vi "Execute Network Operation.vi"(7 "Operation":T1, 8 "error in (no error)":errorcluster, 10 "Message":string, 11 "Listener In.lvclass":refnum<class "Listener.lvclass">) -> (0 "error out":errorcluster, 3 "Listener Out.lvclass":refnum<class "Listener.lvclass">)   [LabVIEW 2023, in "Listener.lvclass"]
doc: "Reads/Writes data using the specified protocol.\nInput: \nListener Object\nMessage: The \"packet\" which will be sent through the selected protocol\nOpeartion: Read/Write operation on the specified protocol"
uses:
  Listener.lvclass
  Protocols.lvlib
  Constants.vi
  ListenerClassControls/Operation.ctl
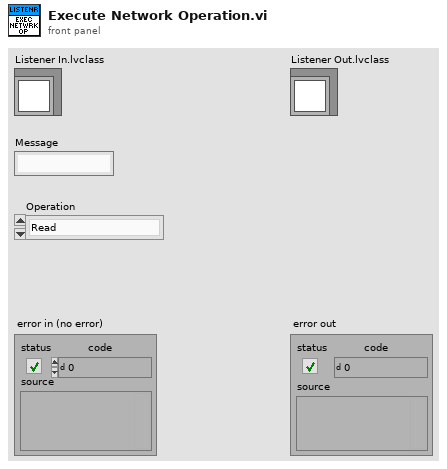
[diagram p1: front panel]
types:
  T1 = typedef "Listener.lvclass/Operation.ctl" = enum16{"Read", "Write"}
  T2 = enum16{"Standard", "Buffered", "CRLF", "Immediate"}
  T3 = typedef "Listener.lvclass/Protocol.ctl" = enum16{"RS-XXX", "AK RS-XXX", "VISA", "TCPIP", "AK TCPIP", "UDP", "GPIB ConvBox"}
  T4 = typedef "Listener.lvclass/UDP Data Structure.ctl" = cluster{"UDP connection ID":refnum<k16>, "Local Address":string, "Local Port":u16, "Target IP Address":string, "Target Port":u16, "Data":string}
  T5 = typedef "Listener.lvclass/TCP Data Structure.ctl" = cluster{"TCP|IP connection ID":refnum<k5>, "IP Address":string, "Port":u16, "Data":string}
  T6 = typedef "Listener.lvclass/AK TCP Data Structure.ctl" = cluster{"TCP|IP connection ID":refnum<k5>, "IP Address":string, "Port":u16, "Data":string, "Current Command Code":string}
  T7 = typedef "Listener.lvclass/VISA Data Structure.ctl" = cluster{"Data Length":u32, "Data":string}
  T8 = typedef "Listener.lvclass/RS-xxx Data Structure.ctl" = cluster{"Virtual COM Port Settings 1":cluster{"Port":string, "Baud Rate":u32, "Data Bits":u16, "Parity":enum16{"None", "Odd", "Even", "Mark", "Space"}, "Stop Bits":u16, "Flow Control":u16, "XON":enum16{"NUL", "SOH", "STX", "ETX", "EOT", "ENQ", "ACK", "BEL", "BS", "HT", "LF", "VT", "FF", "CR", "SO", "SI", "DLE", "DC1", "DC2", "DC3", "DC4", "NAK", "SYN", "ETB", "CAN", "EM", "SUB", "ESC", "FS", "GS", "RS", "US", "SP", "!", "\"", "#", "$", "%", "&", "'", "(", ")", "*", "+", ",", "- (-)", ".", "/", "0", "1", "2", "3", "4", "5", "6", "7", "8", "9", ":", ";", "<", "=", ">", "?", "@", "A", "B", "C", "D", "E", "F", "G", "H", "I", "J", "K", "L", "M", "N", "O", "P", "Q", "R", "S", "T", "U", "V", "W", "X", "Y", "Z", "[", "\\", "]", "^", "_", "`", "a", "b", "c", "d", "e", "f", "g", "h", "i", "j", "k", "l", "m", "n", "o", "p", "q", "r", "s", "t", "u", "v", "w", "x", "y", "z", "{", "|", "}", "~"}, "XOFF":enum16{"NUL", "SOH", "STX", "ETX", "EOT", "ENQ", "ACK", "BEL", "BS", "HT", "LF", "VT", "FF", "CR", "SO", "SI", "DLE", "DC1", "DC2", "DC3", "DC4", "NAK", "SYN", "ETB", "CAN", "EM", "SUB", "ESC", "FS", "GS", "RS", "US", "SP", "!", "\"", "#", "$", "%", "&", "'", "(", ")", "*", "+", ",", "- (-)", ".", "/", "0", "1", "2", "3", "4", "5", "6", "7", "8", "9", ":", ";", "<", "=", ">", "?", "@", "A", "B", "C", "D", "E", "F", "G", "H", "I", "J", "K", "L", "M", "N", "O", "P", "Q", "R", "S", "T", "U", "V", "W", "X", "Y", "Z", "[", "\\", "]", "^", "_", "`", "a", "b", "c", "d", "e", "f", "g", "h", "i", "j", "k", "l", "m", "n", "o", "p", "q", "r", "s", "t", "u", "v", "w", "x", "y", "z", "{", "|", "}", "~"}, "End Read on Termination Character":bool, "End Write on Termination Character":bool, "Termination Character":u8}, "Virtual COM Port Settings 2":cluster{"Port":string, "Baud Rate":u32, "Data Bits":u16, "Parity":enum16{"None", "Odd", "Even", "Mark", "Space"}, "Stop Bits":u16, "Flow Control":u16, "XON":enum16{"NUL", "SOH", "STX", "ETX", "EOT", "ENQ", "ACK", "BEL", "BS", "HT", "LF", "VT", "FF", "CR", "SO", "SI", "DLE", "DC1", "DC2", "DC3", "DC4", "NAK", "SYN", "ETB", "CAN", "EM", "SUB", "ESC", "FS", "GS", "RS", "US", "SP", "!", "\"", "#", "$", "%", "&", "'", "(", ")", "*", "+", ",", "- (-)", ".", "/", "0", "1", "2", "3", "4", "5", "6", "7", "8", "9", ":", ";", "<", "=", ">", "?", "@", "A", "B", "C", "D", "E", "F", "G", "H", "I", "J", "K", "L", "M", "N", "O", "P", "Q", "R", "S", "T", "U", "V", "W", "X", "Y", "Z", "[", "\\", "]", "^", "_", "`", "a", "b", "c", "d", "e", "f", "g", "h", "i", "j", "k", "l", "m", "n", "o", "p", "q", "r", "s", "t", "u", "v", "w", "x", "y", "z", "{", "|", "}", "~"}, "XOFF":enum16{"NUL", "SOH", "STX", "ETX", "EOT", "ENQ", "ACK", "BEL", "BS", "HT", "LF", "VT", "FF", "CR", "SO", "SI", "DLE", "DC1", "DC2", "DC3", "DC4", "NAK", "SYN", "ETB", "CAN", "EM", "SUB", "ESC", "FS", "GS", "RS", "US", "SP", "!", "\"", "#", "$", "%", "&", "'", "(", ")", "*", "+", ",", "- (-)", ".", "/", "0", "1", "2", "3", "4", "5", "6", "7", "8", "9", ":", ";", "<", "=", ">", "?", "@", "A", "B", "C", "D", "E", "F", "G", "H", "I", "J", "K", "L", "M", "N", "O", "P", "Q", "R", "S", "T", "U", "V", "W", "X", "Y", "Z", "[", "\\", "]", "^", "_", "`", "a", "b", "c", "d", "e", "f", "g", "h", "i", "j", "k", "l", "m", "n", "o", "p", "q", "r", "s", "t", "u", "v", "w", "x", "y", "z", "{", "|", "}", "~"}, "End Read on Termination Character":bool, "End Write on Termination Character":bool, "Termination Character":u8}, "Data":string, "Data Length":u32}
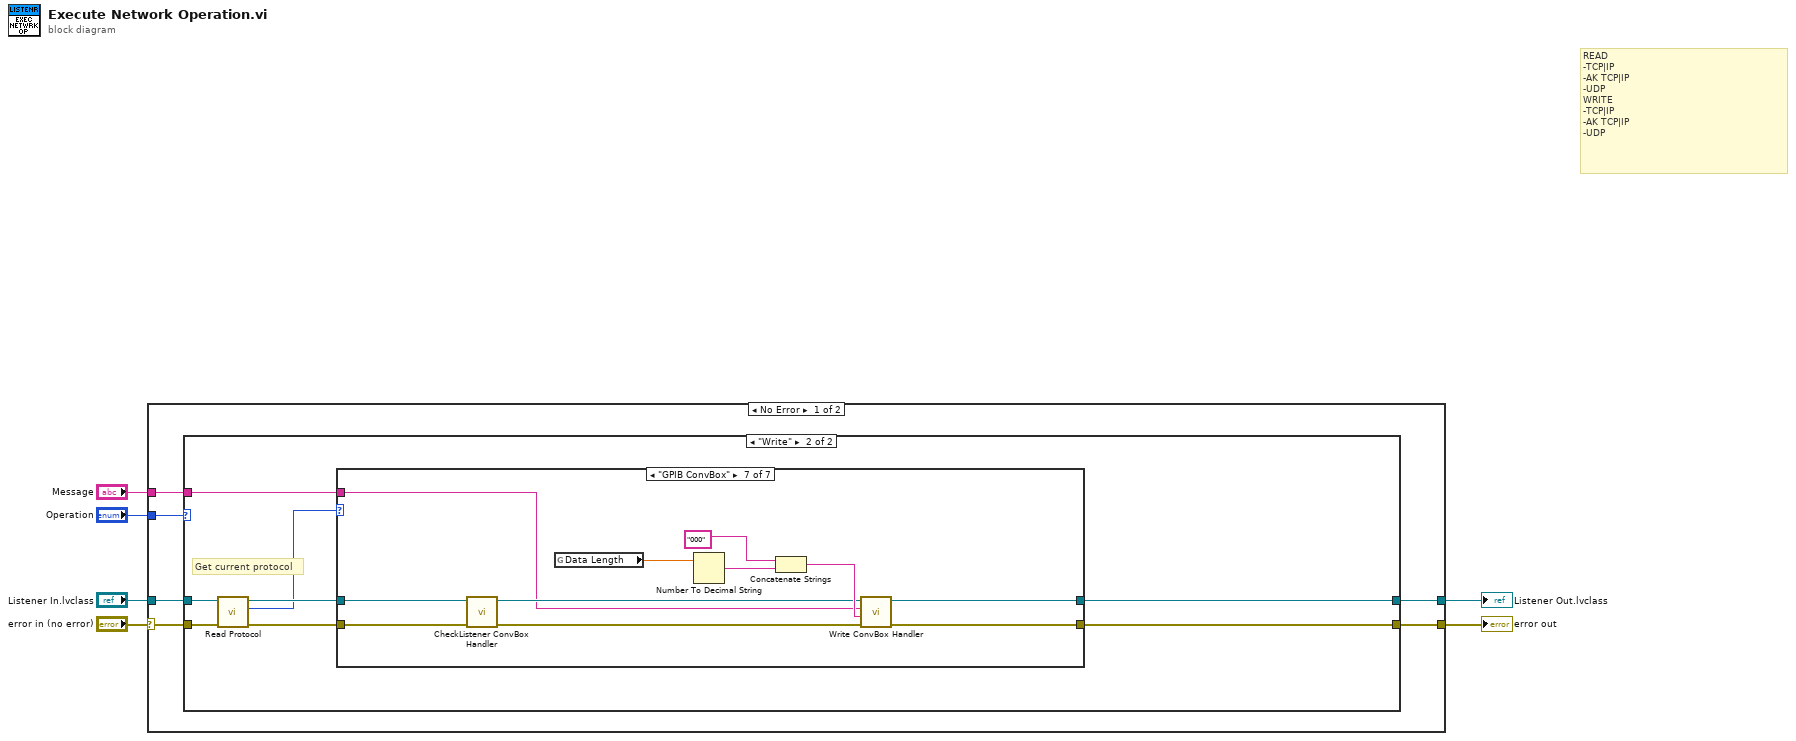
[diagram p0: block diagram]
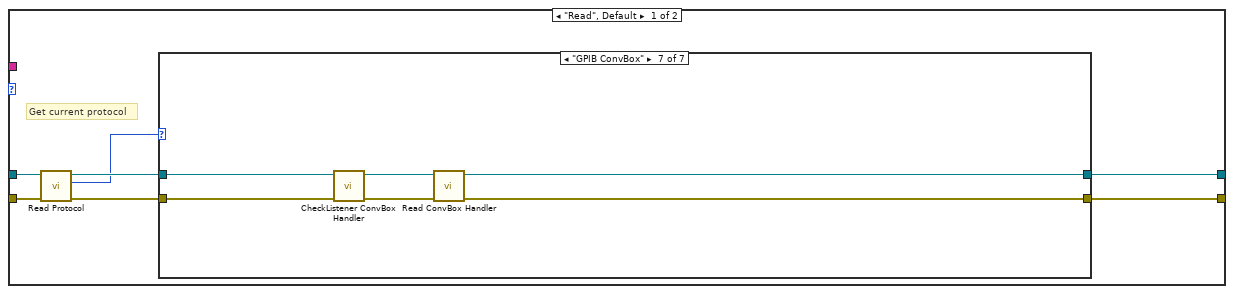
[diagram p2: hidden frame]
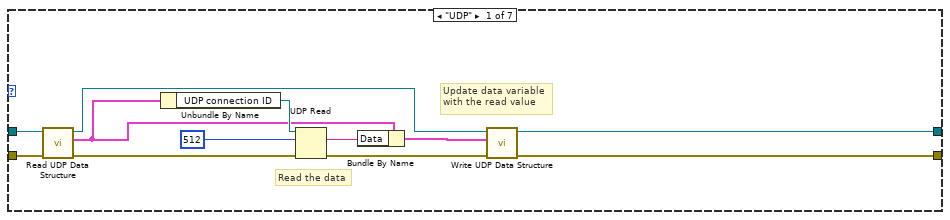
[diagram p3: hidden frame]
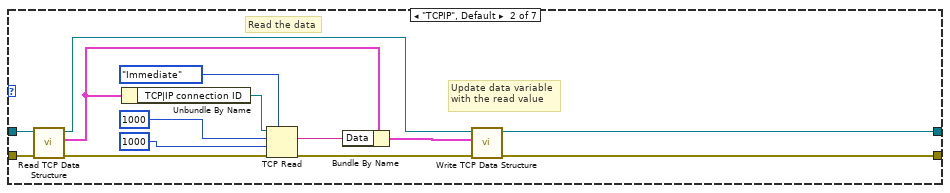
[diagram p4: hidden frame]
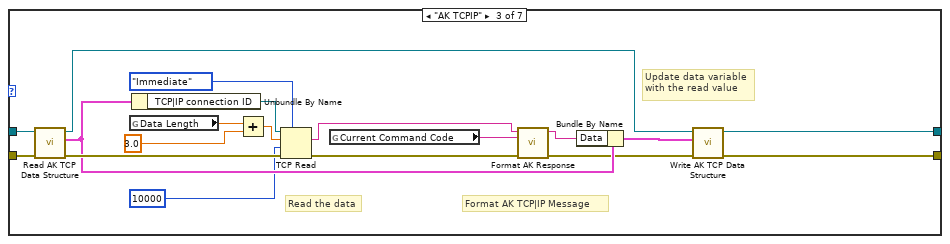
[diagram p5: hidden frame]
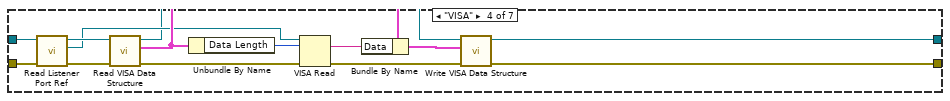
[diagram p6: hidden frame]
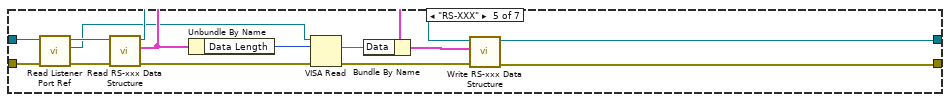
[diagram p7: hidden frame]
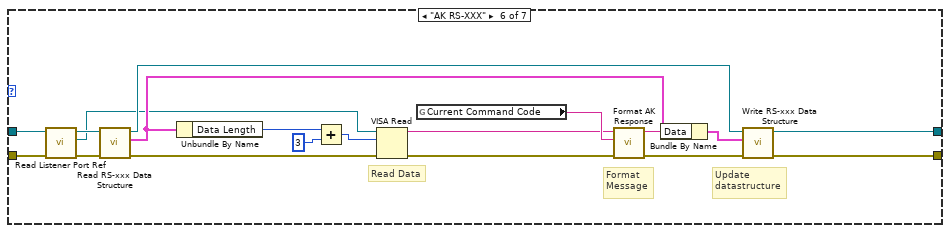
[diagram p8: hidden frame]
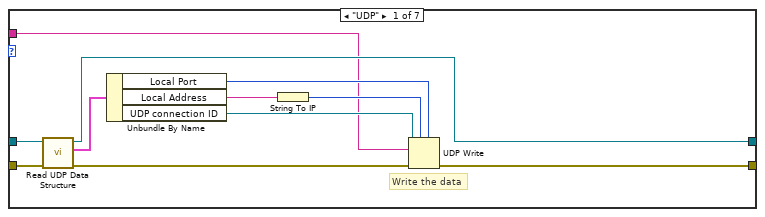
[diagram p9: hidden frame]
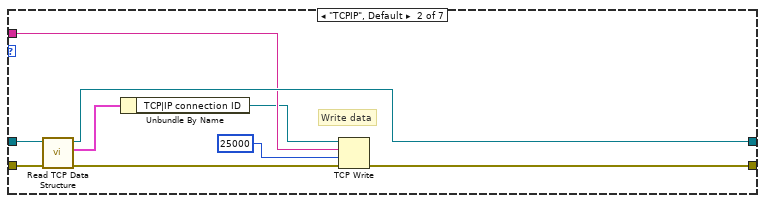
[diagram p10: hidden frame]
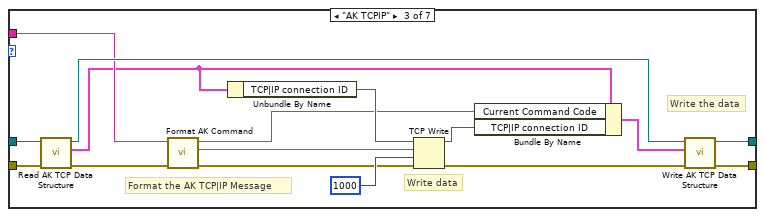
[diagram p11: hidden frame]
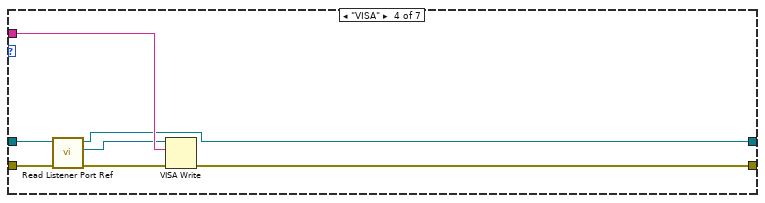
[diagram p12: hidden frame]
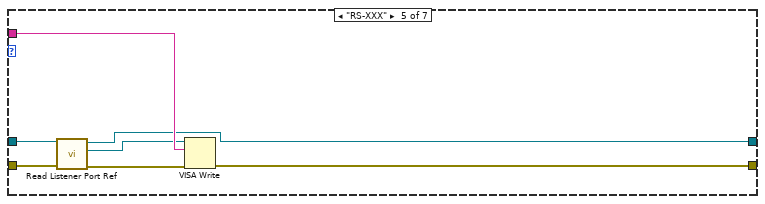
[diagram p13: hidden frame]
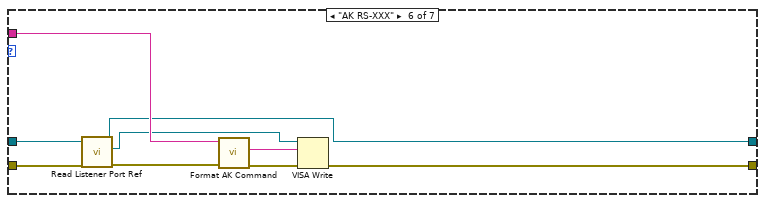
[diagram p14: hidden frame]
diagram:
  # "READ\n-TCP|IP\n-AK TCP|IP\n-UDP\nWRITE\n-TCP|IP\n-AK TCP|IP\n-UDP"
  n1 = case shown="No Error" "error in (no error)" {
    selector: "error in (no error)" -> [w9 w196]
    tunnel: "Listener In.lvclass" -> [w12 w197]
    tunnel: [w11 w196] -> w5
    tunnel: [w10 w197] -> w4
    tunnel: "Operation" -> [w8 _]
    tunnel: "Message" -> [w7 _]
    frame No Error {
      n2 = case shown="\"Write\"" w8 {
        tunnel: w9 -> [w19 w123]
        tunnel: w12 -> [w18 w120]
        tunnel: [w15 w124] -> w11
        tunnel: [w14 w125] -> w10
        tunnel: w7 -> [_ w118]
        frame "Read", Default {
          # "Get current protocol"
          n3 = call-dynamic "Read Protocol.vi"("error in (no error)"=w19, "Listener in"=w18) -> ("error out"=w17:errorcluster, "Protocol"=w13:T3, "Listener out"=w16:refnum<class "Listener.lvclass">)  [unwired: 7 in]
          n4 = case shown="\"GPIB ConvBox\"" w13 {
            tunnel: w17 -> [w31 w45 w53 w70 w82 w96 w113]
            tunnel: w16 -> [w30 w44 w54 w68 w83 w97 w115]
            tunnel: [w28 w42 w51 w75 w88 w110 w116] -> w14
            tunnel: [w29 w43 w52 w77 w87 w108 w117] -> w15
            frame "UDP" {
              # "Read the data"
              # "Update data variable\nwith the read value"
              n5 = call-dynamic "Read UDP Data Structure.vi"("error in (no error)"=w31, "Listener in"=w30) -> ("error out"=w27:errorcluster, "UDP Data Structure"=w24:T4, "Listener out"=w21:refnum<class "Listener.lvclass">)  [unwired: 7 in]
              n6 = Unbundle By Name(w24) -> ("UDP connection ID"=w25:refnum<k16>)
              n7 = UDP Read(connection ID=w25, max size (548)=512, 8:w27) -> (data out=w23:string, error out=w22:errorcluster)  [unwired: 1 in, 3 out]
              n8 = Bundle By Name(cluster=w24, "Data"=w23) -> (w20:T4)
              n9 = call-dynamic "Write UDP Data Structure.vi"("error in (no error)"=w22, "UDP Data Structure"=w20, "Listener in"=w21) -> ("error out"=w29:errorcluster, "Listener out"=w28:refnum<class "Listener.lvclass">)  [unwired: 7 in]
            }
            frame "TCPIP", Default {
              # "Update data variable\nwith the read value"
              # "Read the data"
              n10 = call-dynamic "Read TCP Data Structure.vi"("error in (no error)"=w45, "Listener in"=w44) -> ("error out"=w40:errorcluster, "TCP|IP Data Structure"=w39:T5, "Listener out"=w35:refnum<class "Listener.lvclass">)  [unwired: 7 in]
              n11 = Unbundle By Name(w39) -> ("TCP|IP connection ID"=w34:refnum<k5>)
              n12 = TCP Read(connection ID=w34, bytes to read=1000, error in (no error)=w40, 7:T2."Immediate" ("mode (standard)"), 9:1000 ("timeout ms (25000)")) -> (data out=w38:string, error out=w36:errorcluster)  [unwired: 1 out]
              n13 = Bundle By Name(cluster=w39, "Data"=w38) -> (w37:T5)
              n14 = call-dynamic "Write TCP Data Structure.vi"("error in (no error)"=w36, "TCP|IP Data Structure"=w37, "Listener in"=w35) -> ("error out"=w43:errorcluster, "Listener out"=w42:refnum<class "Listener.lvclass">)  [unwired: 7 in]
            }
            frame "AK TCPIP" {
              # "Format AK TCP|IP Message"
              # "Update data variable\nwith the read value"
              # "Read the data"
              n15 = call-dynamic "Read AK TCP Data Structure.vi"("error in (no error)"=w53, "Listener in"=w54) -> ("error out"=w63:errorcluster, "TCP|IP Data Structure"=w61:T6, "Listener out"=w57:refnum<class "Listener.lvclass">)  [unwired: 7 in]
              n16 = global read "Constants.vi" "Data Length"() -> (w50:dbl)
              n17 = Unbundle By Name(w61) -> ("TCP|IP connection ID"=w64:refnum<k5>)
              n18 = Add(x=w50, y=3.0) -> (x+y=w48:dbl)
              n19 = TCP Read(connection ID=w64, bytes to read=w48, error in (no error)=w63, 7:T2."Immediate" ("mode (standard)"), 9:10000 ("timeout ms (25000)")) -> (data out=w46:string, error out=w62:errorcluster)  [unwired: 1 out]
              n20 = global read "Constants.vi" "Current Command Code"() -> (w47:string)
              n21 = call "Format AK Response.vi"("error in (no error)"=w62, "Current Command Code"=w47, "Response"=w46) -> ("error out"=w59:errorcluster, "Data"=w60:string)  [unwired: 7 in]
              n22 = Bundle By Name(cluster=w61, "Data"=w60) -> (w58:T6)
              n23 = call-dynamic "Write AK TCP Data Structure.vi"("error in (no error)"=w59, "TCP|IP Data Structure"=w58, "Listener in"=w57) -> ("error out"=w52:errorcluster, "Listener out"=w51:refnum<class "Listener.lvclass">)  [unwired: 7 in]
            }
            frame "VISA" {
              n24 = call "Read Listener Port Ref.vi"("error in (no error)"=w70, "Listener in"=w68) -> ("error out"=w69:errorcluster, "Listener Port Ref"=w66:refnum<visa-resource-name>, "Listener out"=w67:refnum<class "Listener.lvclass">)  [unwired: 7 in]
              n25 = call-dynamic "Read VISA Data Structure.vi"("error in (no error)"=w69, "Listener in"=w67) -> ("error out"=w71:errorcluster, "VISA Data Structure"=w78:T7, "Listener out"=w65:refnum<class "Listener.lvclass">)  [unwired: 7 in]
              n26 = Unbundle By Name(w78) -> ("Data Length"=w72:u32)
              n27 = VISA Read(VISA resource name=w66, byte count=w72, error in (no error)=w71) -> (read buffer=w73:string, error out=w74:errorcluster)  [unwired: 2 out]
              n28 = Bundle By Name(cluster=w78, "Data"=w73) -> (w76:T7)
              n29 = call-dynamic "Write VISA Data Structure.vi"("error in (no error)"=w74, "VISA Data Structure"=w76, "Listener in"=w65) -> ("error out"=w77:errorcluster, "Listener out"=w75:refnum<class "Listener.lvclass">)  [unwired: 7 in]
            }
            frame "RS-XXX" {
              n30 = call "Read Listener Port Ref.vi"("error in (no error)"=w82, "Listener in"=w83) -> ("error out"=w81:errorcluster, "Listener Port Ref"=w79:refnum<visa-resource-name>, "Listener out"=w80:refnum<class "Listener.lvclass">)  [unwired: 7 in]
              n31 = call-dynamic "Read RS-xxx Data Structure.vi"("error in (no error)"=w81, "Listener in"=w80) -> ("error out"=w85:errorcluster, "RS-xxx Data Structure"=w86:T8, "Listener out"=w90:refnum<class "Listener.lvclass">)  [unwired: 7 in]
              n32 = Unbundle By Name(w86) -> ("Data Length"=w84:u32)
              n33 = VISA Read(VISA resource name=w79, byte count=w84, error in (no error)=w85) -> (read buffer=w92:string, error out=w89:errorcluster)  [unwired: 2 out]
              n34 = Bundle By Name(cluster=w86, "Data"=w92) -> (w91:T8)
              n35 = call-dynamic "Write RS-xxx Data Structure.vi"("error in (no error)"=w89, "RS-xxx Data Structure"=w91, "Listener in"=w90) -> ("error out"=w87:errorcluster, "Listener out"=w88:refnum<class "Listener.lvclass">)  [unwired: 7 in]
            }
            frame "AK RS-XXX" {
              # "Update \ndatastructure"
              # "Format \nMessage"
              # "Read Data"
              n36 = call "Read Listener Port Ref.vi"("error in (no error)"=w96, "Listener in"=w97) -> ("error out"=w95:errorcluster, "Listener Port Ref"=w93:refnum<visa-resource-name>, "Listener out"=w94:refnum<class "Listener.lvclass">)  [unwired: 7 in]
              n37 = call-dynamic "Read RS-xxx Data Structure.vi"("error in (no error)"=w95, "Listener in"=w94) -> ("error out"=w109:errorcluster, "RS-xxx Data Structure"=w111:T8, "Listener out"=w107:refnum<class "Listener.lvclass">)  [unwired: 7 in]
              n38 = Unbundle By Name(w111) -> ("Data Length"=w106:u32)
              n39 = Add(x=w106, y=u32 3) -> (x+y=w98:u32)
              n40 = VISA Read(VISA resource name=w93, byte count=w98, error in (no error)=w109) -> (read buffer=w101:string, error out=w100:errorcluster)  [unwired: 2 out]
              n41 = global read "Constants.vi" "Current Command Code"() -> (w103:string)
              n42 = call "Format AK Response.vi"("error in (no error)"=w100, "Current Command Code"=w103, "Response"=w101) -> ("error out"=w102:errorcluster, "Data"=w105:string)  [unwired: 7 in]
              n43 = Bundle By Name(cluster=w111, "Data"=w105) -> (w104:T8)
              n44 = call-dynamic "Write RS-xxx Data Structure.vi"("error in (no error)"=w102, "RS-xxx Data Structure"=w104, "Listener in"=w107) -> ("error out"=w108:errorcluster, "Listener out"=w110:refnum<class "Listener.lvclass">)  [unwired: 7 in]
            }
            frame "GPIB ConvBox" {
              n45 = call "CheckListener ConvBox Handler.vi"("error in (no error)"=w113, "Listener in"=w115) -> ("error out"=w112:errorcluster, "Listener out"=w114:refnum<class "Listener.lvclass">)  [unwired: 8 in]
              n46 = call "Read ConvBox Handler.vi"("error in (no error)"=w112, "Listener in"=w114) -> ("error out"=w117:errorcluster, "Listener out"=w116:refnum<class "Listener.lvclass">)  [unwired: 8 in]
            }
          }
        }
        frame "Write" {
          # "Get current protocol"
          n47 = call-dynamic "Read Protocol.vi"("error in (no error)"=w123, "Listener in"=w120) -> ("error out"=w122:errorcluster, "Protocol"=w119:T3, "Listener out"=w121:refnum<class "Listener.lvclass">)  [unwired: 7 in]
          n48 = case shown="\"GPIB ConvBox\"" w119 {
            tunnel: [w133 w145 w149 w162 w169 w177 w195] -> w125
            tunnel: [w134 w144 w148 w167 w175 w183 w194] -> w124
            tunnel: w121 -> [w135 w142 w147 w166 w172 w179 w188]
            tunnel: w122 -> [w136 w143 w150 w165 w173 w180 w187]
            tunnel: w118 -> [w126 w141 w151 w168 w174 w184 w185]
            frame "UDP" {
              # "Write the data"
              n49 = call-dynamic "Read UDP Data Structure.vi"("error in (no error)"=w136, "Listener in"=w135) -> ("error out"=w130:errorcluster, "UDP Data Structure"=w132:T4, "Listener out"=w133:refnum<class "Listener.lvclass">)  [unwired: 7 in]
              n50 = Unbundle By Name(w132) -> ("Local Port"=w129:u16, "Local Address"=w128:string, "UDP connection ID"=w131:refnum<k16>)
              n51 = String To IP(1:w128) -> (0:w127:u32)
              n52 = UDP Write(address=w127, port or service name=w129, connection ID=w131, data in=w126, 8:w130) -> (error out=w134:errorcluster)  [unwired: 1 in, 1 out]
            }
            frame "TCPIP", Default {
              # "Write data"
              n53 = call-dynamic "Read TCP Data Structure.vi"("error in (no error)"=w143, "Listener in"=w142) -> ("error out"=w137:errorcluster, "TCP|IP Data Structure"=w139:T5, "Listener out"=w145:refnum<class "Listener.lvclass">)  [unwired: 7 in]
              n54 = Unbundle By Name(w139) -> ("TCP|IP connection ID"=w140:refnum<k5>)
              n55 = TCP Write(connection ID=w140, data in=w141, error in (no error)=w137, 9:25000 ("timeout ms (25000)")) -> (error out=w144:errorcluster)  [unwired: 2 out]
            }
            frame "AK TCPIP" {
              # "Format the AK TCP|IP Message"
              # "Write the data"
              # "Write data"
              n56 = call-dynamic "Read AK TCP Data Structure.vi"("error in (no error)"=w150, "Listener in"=w147) -> ("error out"=w158:errorcluster, "TCP|IP Data Structure"=w146:T6, "Listener out"=w157:refnum<class "Listener.lvclass">)  [unwired: 7 in]
              n57 = call "Format AK Command.vi"("error in (no error)"=w158, "String in"=w151) -> ("error out"=w159:errorcluster, "Command"=w155:string, "Command Code"=w154:string)  [unwired: 7 in]
              n58 = Unbundle By Name(w146) -> ("TCP|IP connection ID"=w161:refnum<k5>)
              n59 = TCP Write(connection ID=w161, data in=w155, error in (no error)=w159, 9:1000 ("timeout ms (25000)")) -> (connection ID out=w153:refnum<k5>, error out=w156:errorcluster)  [unwired: 1 out]
              n60 = Bundle By Name(cluster=w146, "Current Command Code"=w154, "TCP|IP connection ID"=w153) -> (w152:T6)
              n61 = call-dynamic "Write AK TCP Data Structure.vi"("error in (no error)"=w156, "TCP|IP Data Structure"=w152, "Listener in"=w157) -> ("error out"=w148:errorcluster, "Listener out"=w149:refnum<class "Listener.lvclass">)  [unwired: 7 in]
            }
            frame "VISA" {
              n62 = call "Read Listener Port Ref.vi"("error in (no error)"=w165, "Listener in"=w166) -> ("error out"=w164:errorcluster, "Listener Port Ref"=w163:refnum<visa-resource-name>, "Listener out"=w162:refnum<class "Listener.lvclass">)  [unwired: 7 in]
              n63 = VISA Write(VISA resource name=w163, write buffer=w168, error in (no error)=w164) -> (error out=w167:errorcluster)  [unwired: 2 out]
            }
            frame "RS-XXX" {
              n64 = call "Read Listener Port Ref.vi"("error in (no error)"=w173, "Listener in"=w172) -> ("error out"=w171:errorcluster, "Listener Port Ref"=w170:refnum<visa-resource-name>, "Listener out"=w169:refnum<class "Listener.lvclass">)  [unwired: 7 in]
              n65 = VISA Write(VISA resource name=w170, write buffer=w174, error in (no error)=w171) -> (error out=w175:errorcluster)  [unwired: 2 out]
            }
            frame "AK RS-XXX" {
              n66 = call "Read Listener Port Ref.vi"("error in (no error)"=w180, "Listener in"=w179) -> ("error out"=w176:errorcluster, "Listener Port Ref"=w178:refnum<visa-resource-name>, "Listener out"=w177:refnum<class "Listener.lvclass">)  [unwired: 7 in]
              n67 = call "Format AK Command.vi"("error in (no error)"=w176, "String in"=w184) -> ("error out"=w182:errorcluster, "Command"=w181:string)  [unwired: 7 in, 1 out]
              n68 = VISA Write(VISA resource name=w178, write buffer=w181, error in (no error)=w182) -> (error out=w183:errorcluster)  [unwired: 2 out]
            }
            frame "GPIB ConvBox" {
              n69 = call "CheckListener ConvBox Handler.vi"("error in (no error)"=w187, "Listener in"=w188) -> ("error out"=w186:errorcluster, "Listener out"=w189:refnum<class "Listener.lvclass">)  [unwired: 8 in]
              n70 = global read "Constants.vi" "Data Length"() -> (w193:dbl)
              n71 = Number To Decimal String(number=w193) -> (decimal integer string=w192:string)  [unwired: 1 in]
              n72 = Concatenate Strings("000" ("string"), w192) -> (w190:string)
              n73 = call "Write ConvBox Handler.vi"("error in (no error)"=w186, "Data Length"=w190, "Data"=w185, "Listener in"=w189) -> ("error out"=w194:errorcluster, "Listener out"=w195:refnum<class "Listener.lvclass">)  [unwired: 6 in]
            }
          }
        }
      }
    }
    frame Error {
    }
  }
  "Listener Out.lvclass" <- w4
  "error out" <- w5
